vi "Stop Core.vi"(10 "final error code":i32, 11 "Acquisition UI in":refnum<class "Acquisition UI.lvclass">) -> (3 "Acquisition UI out":refnum<class "Acquisition UI.lvclass">)   [LabVIEW 2018, in "Acquisition UI.lvlib" / "Acquisition UI.lvclass"]
doc: "(<B>Filename</B>: Actor Framework.lvlib:Actor.lvclass:Stop Core.vi)\n\nDefines what the actor does before it stops. Use the <B>final error code</B> input to determine whether the actor shut down in response to an error.\n\nBy default, this method passes the Stop message along to all auto-stop nested actors. A descendant class may override this method to define additional behavior, such as shutting down any processes the actor initiated in its override of the Actor Core method."
uses:
  Acquisition UI.lvclass
  <vilib>/ActorFramework/Actor/Actor.lvclass
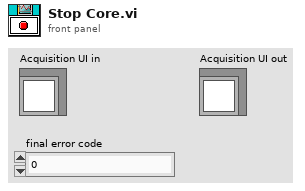
[diagram p1: front panel]
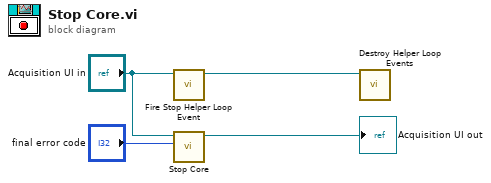
[diagram p0: block diagram]
diagram:
  n1 = call "Fire Stop Helper Loop Event.vi"("Acquisition UI in"="Acquisition UI in") -> ("Acquisition UI out"=w1:refnum<class "Acquisition UI.lvclass">)  [unwired: 10 in]
  n2 = call-parent "Stop Core.vi"("final error code"="final error code", "Actor in"="Acquisition UI in") -> ("Actor out"=→"Acquisition UI out":refnum<class "Acquisition UI.lvclass">)  [unwired: 9 in]
  n3 = call "Destroy Helper Loop Events.vi"("Acquisition UI in"=w1) -> ()  [unwired: 11 in]
